vi "[Global]SeqNumber.vi"() -> ()   [LabVIEW 2015]
panel:
  in  "SeqNumber":i32=200
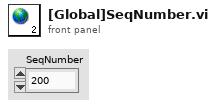
[diagram p1: front panel]
diagram:
